vi "readCursorConfig.vi"(8 "error in (no error)":errorcluster) -> (0 "error out":errorcluster, 3 "Cursor Locations":T1)   [LabVIEW 2019]
uses:
  <vilib>/Utility/config.llb/Read Key (I32).vi
  <vilib>/Utility/config.llb/NI_LVConfig.lvlib
panel:
  out "appended path":path
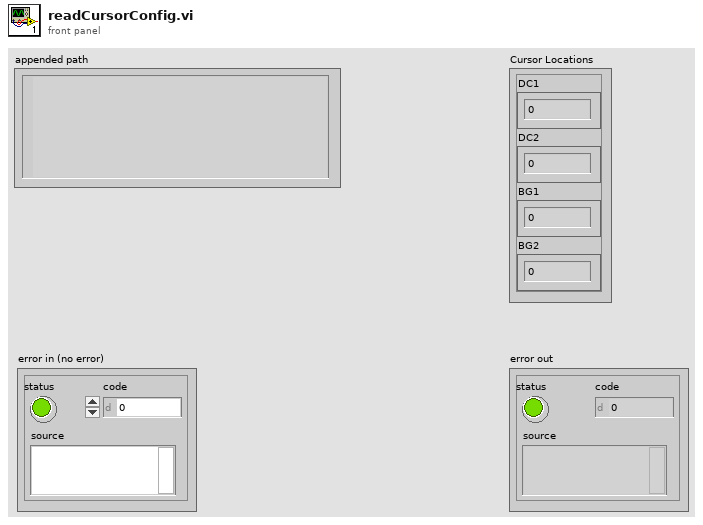
[diagram p1: front panel]
types:
  T1 = cluster{"DC1":i32, "DC2":i32, "BG1":i32, "BG2":i32}
  T2 = typedef "NI_LVConfig.lvlib/Config Data RefNum.ctl" = refnum<k1>
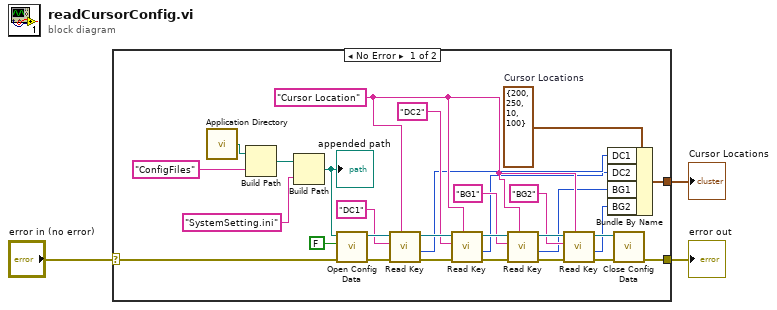
[diagram p0: block diagram]
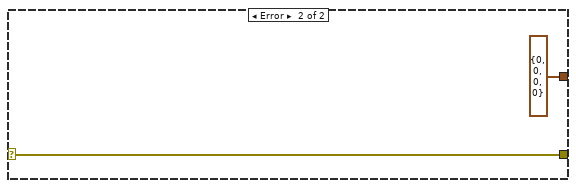
[diagram p2: hidden frame]
diagram:
  n1 = case shown="No Error" "error in (no error)" {
    selector: "error in (no error)" -> [w11 w34]
    tunnel: [w13 w34] -> w3
    tunnel: [w5 T1 {"DC1"=0, "DC2"=0, "BG1"=0, "BG2"=0} ("Cursor Locations")] -> w1
    frame No Error {
      w10 = T1 {"DC1"=200, "DC2"=250, "BG1"=10, "BG2"=100}  # Cursor Locations
      w12 = "Cursor Location" ("section")
      n2 = call <vilib>:"Application Directory.vi"() -> ("Application Directory"=w31:path)
      n3 = Build Path(base path=w31, name or relative path="ConfigFiles") -> (appended path=w29:path)
      n4 = Build Path(base path=w29, name or relative path="SystemSetting.ini") -> (appended path=w4:path)
      "appended path" <- w4
      n5 = call <vilib>:"Open Config Data.vi"("error in (no error)"=w11, "create file if necessary (T)"=FALSE, "configuration file path"=w4) -> ("error out"=w25:errorcluster, "refnum"=w27:T2)  [unwired: 6 in, 1 out]
      n6 = call-poly <vilib>:"Read Key.vi"("section"=w12, "error in (no error)"=w25, "key"="DC1", "refnum"=w27) -> ("error out"=w23:errorcluster, "value"=w9:i32, "refnum out"=w24:T2)  [unwired: 4 in, 1 out]
      n7 = call-poly <vilib>:"Read Key.vi"("section"=w12, "error in (no error)"=w23, "key"="DC2", "refnum"=w24) -> ("error out"=w20:errorcluster, "value"=w8:i32, "refnum out"=w21:T2)  [unwired: 4 in, 1 out]
      n8 = call-poly <vilib>:"Read Key.vi"("section"=w12, "error in (no error)"=w20, "key"="BG1", "refnum"=w21) -> ("error out"=w16:errorcluster, "value"=w7:i32, "refnum out"=w18:T2)  [unwired: 4 in, 1 out]
      n9 = call-poly <vilib>:"Read Key.vi"("section"=w12, "error in (no error)"=w16, "key"="BG2", "refnum"=w18) -> ("error out"=w14:errorcluster, "value"=w6:i32, "refnum out"=w15:T2)  [unwired: 4 in, 1 out]
      n10 = Bundle By Name(cluster=w10, "DC1"=w9, "DC2"=w8, "BG1"=w7, "BG2"=w6) -> (w5:T1)
      n11 = call <vilib>:"Close Config Data.vi"("error in (no error)"=w14, "refnum"=w15) -> ("error out"=w13:errorcluster)  [unwired: 8 in, 1 out]
    }
    frame Error {
    }
  }
  "error out" <- w3
  "Cursor Locations" <- w1
